vi "Calibrate Output.vi"(0 "VISA resource name":refnum<visa-resource-name>, 1 "Unit Address (1)":i16=1, 5 "Output/Retransmit (0: 1A)":i16(ring) items=["1A", "1B", "2A", "2B", "Retransmit 1", "Retransmit 2"], 7 "Calibration (0: 4.000 mA)":u16(ring) items=["4.000 mA", "20.000 mA", "1.000 V", "10.000 V"], 9 "Value (0.0)":dbl format="%.2f", 11 "error in (no error)":errorcluster {"code" format="%.0x"}) -> (4 "VISA resource name out":refnum<visa-resource-name>, 15 "error out":errorcluster {"code" format="%.0x"})   [LabVIEW 2010]
doc: "This VI configures calibrate output and retransmit."
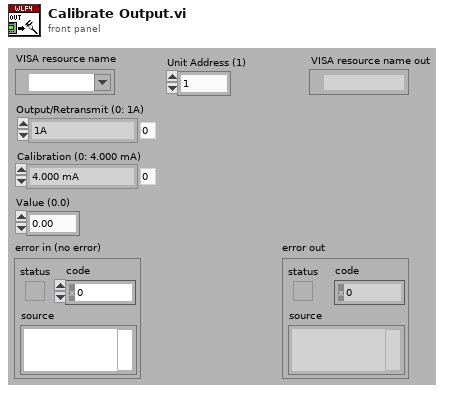
[diagram p1: front panel]
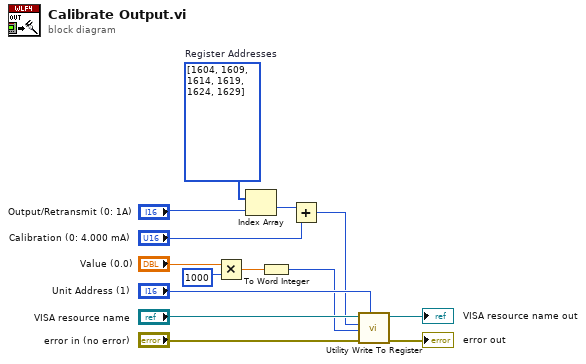
[diagram p0: block diagram]
diagram:
  w9 = i32[] [1604, 1609, 1614, 1619, 1624, 1629]  # Register Addresses
  n1 = Multiply(x="Value (0.0)", y=i16 1000) -> (x*y=w3:dbl)
  n2 = Index Array(array=w9, index="Output/Retransmit (0: 1A)") -> (element=w8:i32)
  n3 = To Word Integer(number=w3) -> (16bit integer=w2:i16)
  n4 = Add(x=w8, y="Calibration (0: 4.000 mA)") -> (x+y=w7:i32)
  n5 = call "Utility Write To Register.vi"("Unit Address (1)"="Unit Address (1)", "error in (no error)"="error in (no error)", "Data (0)"=w2, "Register Address (0)"=w7, "VISA resource name"="VISA resource name") -> ("error out"=→"error out":errorcluster, "VISA resource name out"=→"VISA resource name out":refnum<visa-resource-name>)  [unwired: 5 in]
